vi "Do.vi"(8 "error in (no error)":errorcluster, 10 "Actor in":refnum<class "Actor.lvclass">, 11 "Open FrontPanel Msg":refnum<class "Open FrontPanel Msg.lvclass">) -> (0 "error out":errorcluster, 2 "Actor out":refnum<class "Actor.lvclass">)   [LabVIEW 2017, in "Task Setting Editor.lvlib" / "Open FrontPanel Msg.lvclass"]
doc: "This VI delivers the message to the actor by calling the appropriate method(s) on the actor."
uses:
  Open FrontPanel Msg.lvclass
  <vilib>/ActorFramework/Actor/Actor.lvclass
  Task Setting Editor/Task Setting Editor.lvclass
  Applications/National Instruments/LabVIEW 2017 64-bit/vi.lib/ActorFramework/Actor/Actor.lvclass
  Open FrontPanel Msg.lvclass/Open FrontPanel Msg.ctl
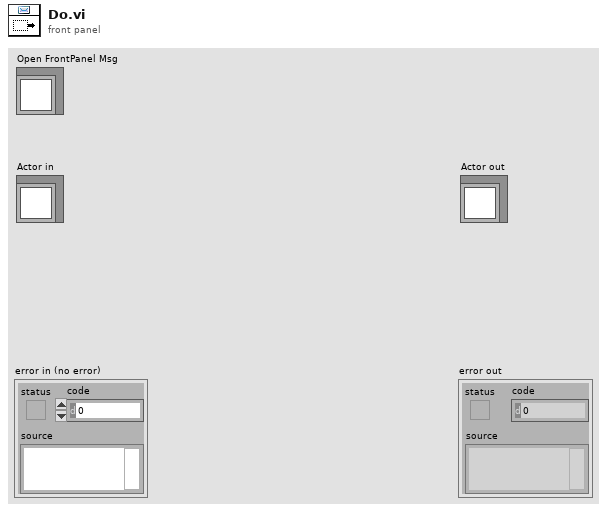
[diagram p1: front panel]
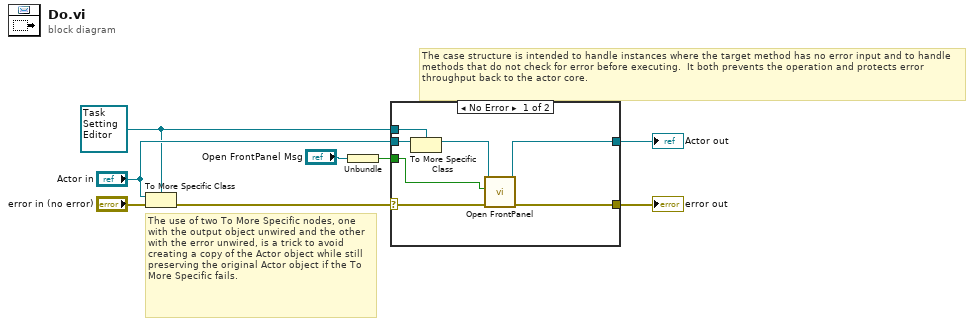
[diagram p0: block diagram]
diagram:
  w2 = refnum<class "Task Setting Editor.lvclass"> refnum ("Actor in")
  # "The use of two To More Specific nodes, one with the output object unwired and the other with the error unwired, is a trick to avoid creating a copy of the Actor object while still preserving the original Actor object if the To More Specific fails."
  # "The case structure is intended to handle instances where the target method has no error input and to handle methods that do not check for error before executing.  It both prevents the operation and protects error throughput back to the actor core."
  n1 = To More Specific Class(target class=w2, reference="Actor in", error in="error in (no error)") -> (error out=w6:errorcluster)  [unwired: 1 out]
  n2 = Unbundle("Open FrontPanel Msg") -> (w1:bool)
  n3 = case shown="No Error" w6 {
    selector: w6 -> [w14 w17]
    tunnel: [w15 w17] -> w5
    tunnel: [w10 w16] -> w4
    tunnel: "Actor in" -> [w13 w16]
    tunnel: w2 -> [w12 _]
    tunnel: w1 -> [w9 _]
    frame No Error {
      n4 = To More Specific Class(target class=w12, reference=w13) -> (specific class reference=w11:refnum<class "Task Setting Editor.lvclass">)  [unwired: 1 in, 1 out]
      n5 = call "Open FrontPanel.vi"("Task Setting Editor in"=w11, "Open"=w9, "error in (no error)"=w14) -> ("Task Setting Editor out"=w10:refnum<class "Task Setting Editor.lvclass">, "error out"=w15:errorcluster)  [unwired: 6 in]
    }
    frame Error {
      # "If type check fails, pass the original object out again."
    }
  }
  "error out" <- w5
  "Actor out" <- w4
